vi "Flat_sequence_and_case_structure.vi"() -> ()   [LabVIEW 2017]
panel:
  out "n'th Fibonacci number":dbl
  in  "n":dbl
  out "number (0 to 1)":dbl
  in  "stop":bool
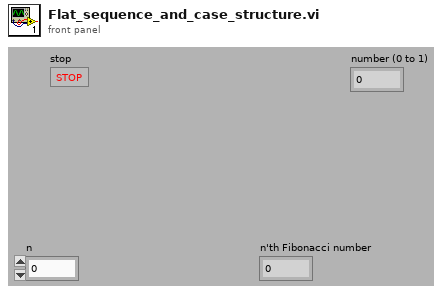
[diagram p1: front panel]
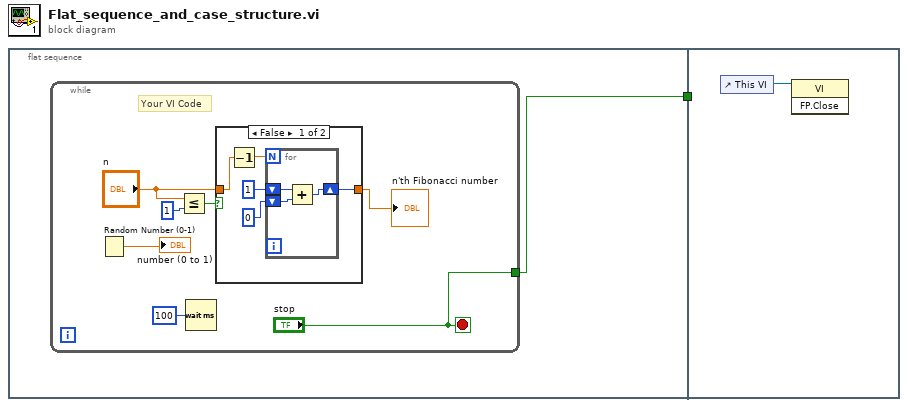
[diagram p0: block diagram]
diagram:
  n1 = flat-sequence {
    tunnel: [w2] -> w1
    tunnel: w1 -> [_]
    frame #0 {
      n2 = while {
        tunnel: ["stop"] -> w2
        stop <- "stop" stop-if-true
        # "Your VI Code"
        n3 = Random Number (0-1)() -> (number: 0 to 1=→"number (0 to 1)":dbl)
        n4 = Less Or Equal?(x="n", y=1) -> (x <= y?=w4:bool)
        n5 = Wait (ms)(milliseconds to wait=u32 100) -> ()  [unwired: 1 out]
        n6 = case shown="False" w4 {
          tunnel: "n" -> [w12 w18]
          tunnel: [w10 w18] -> w3
          frame False {
            n7 = Decrement(x=w12) -> (x-1=w11:dbl)
            n8 = for {
              N: w11 -> [_]
              shift-right: [w15] -> w10
              shift-left: 1 -> [w17]
              shift-left: 0 -> [w16]
              n9 = Add(x=w17, y=w16) -> (x+y=w15:i32)
            }
          }
          frame True {
          }
        }
        "n'th Fibonacci number" <- w3
      }
    }
    frame #1 {
      n10 = control-ref of="This VI"() -> (w19:refnum<vi>)
      n11 = invoke class="VI" method="FP.Close"(reference=w19) -> ()  [unwired: 2 in, 3 out]
    }
  }
